vi "8HP_Channels.vi"(1 "Analysis Info cluster":T2[](array[typedef]) {"Sync Delay Time (s)" format="%.4f"; "Sd Error in Variance" format="%.2f"; "Skew_u" format="%.2f"; "% u'/U" format="%.2f"; "Sd Error in Mean" format="%.2f"; "Kurt_u" format="%.2f"; "u^4" format="%.2f"; "u^3" format="%.2f"; "U" format="%.2f"; "u^2" format="%.2f"}) -> (0 "8HP Info":T1(array[cluster]))   [LabVIEW 2018]
uses:
  Controls/Analysis_info_cluster.ctl
  Controls/Inst_type.ctl
  Controls/Instrument_Array.ctl
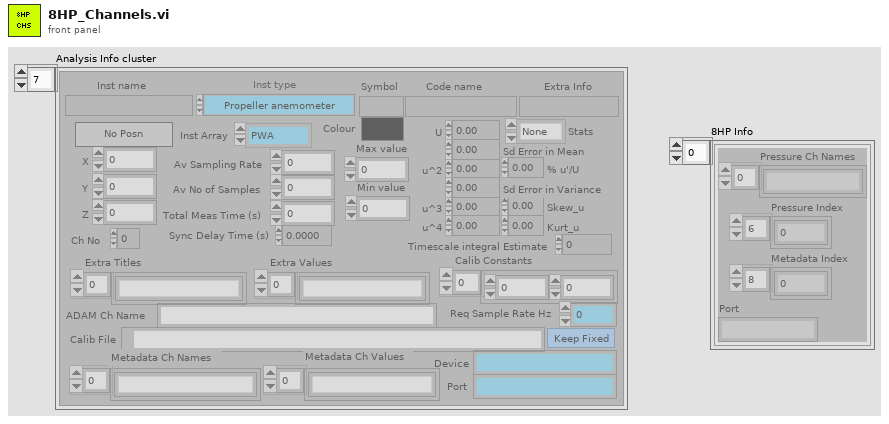
[diagram p1: front panel]
types:
  T1 = cluster{"Pressure Ch Names":string[], "Pressure Index":i32[], "Metadata Index":i32[], "Port":string}[]
  T2 = typedef "Analysis_info_cluster.ctl" = cluster{"Colour":u32, "Inst type":T3, "Inst name":string, "Symbol":string, "Code name":string, "Extra Info":string, "Inst Array":T4, "Extra Titles":string[], "Extra Values":string[], "U":dbl, "u^2":dbl, "u^3":dbl, "u^4":dbl, "Skew_u":dbl, "Kurt_u":dbl, "Sd Error in Mean":dbl, "% u'/U":dbl, "X":dbl, "Y":dbl, "Z":dbl, "Timescale integral Estimate":dbl, "Sd Error in Variance":dbl, "Calib File":path, "Calib Constants":dbl[], "Output Position":bool, "Stats":enum16{"None", "Basic", "Full"}, "Av Sampling Rate":dbl, "Av No of Samples":dbl, "Total Meas Time (s)":dbl, "ADAM Ch Name":string, "Max value":dbl, "Min value":dbl, "Req Sample Rate Hz":dbl, "Sync Delay Time (s)":dbl, "Ch No":i16, "Device":string, "Use Latest Calib":bool, "Port":string, "Metadata Ch Names":string[], "Metadata Ch Values":string[]}
  T3 = typedef "Inst_type.ctl" = enum16{"Propeller anemometer", "Raw voltage", "Pressure Transducer", "Pitot-static tube", "Preston tube", "Hot wire", "Cross wire 1", "Cross wire 2", "Generic Linear", "Generic Polynomial", "Generic BackPoly", "Fast FID", "Thermocouple", "Cold wire", "Pulsed Wire", "LDA Vel", "LDA Tran time", "LDA Arr time", "Microphone"}
  T4 = typedef "Instrument_Array.ctl" = enum16{"PWA", "LDA", "Analogue"}
  T5 = cluster{"Pressure Ch Names":string[], "Pressure Index":i32[], "Metadata Index":i32[], "Port":string}
  T6 = typedef "Device ID port info.ctl" = cluster{"Ch No":i16[], "Req Sampling Rate":dbl[], "Port":string, "Index":i32[]}
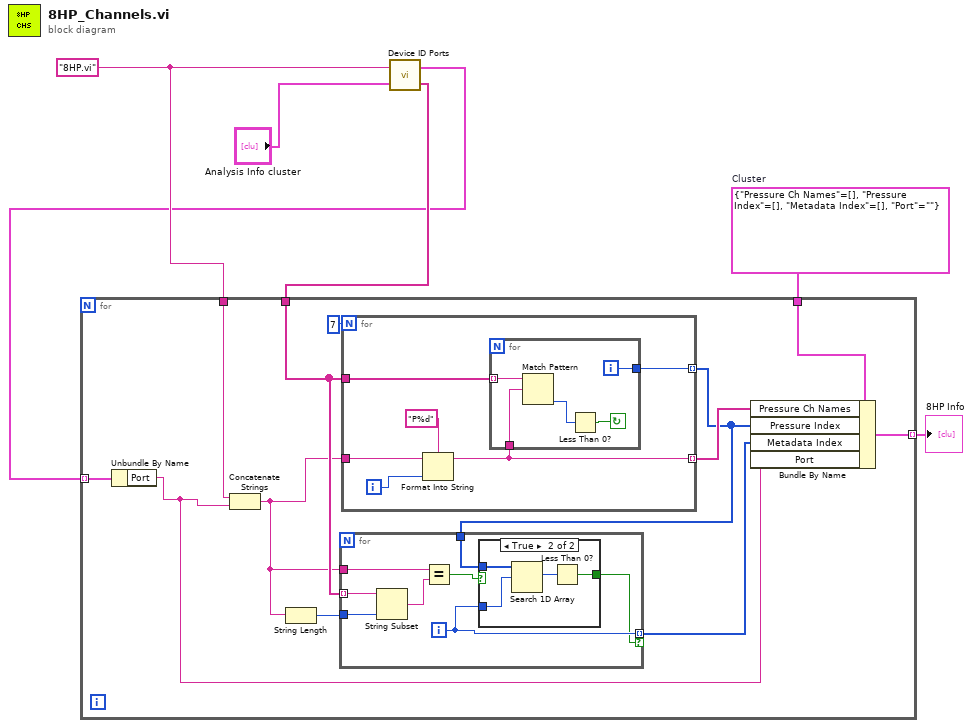
[diagram p0: block diagram]
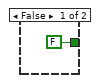
[diagram p2: hidden frame]
diagram:
  w3 = T5 {"Pressure Ch Names"=[], "Pressure Index"=[], "Metadata Index"=[], "Port"=""}  # Cluster
  w5 = "8HP.vi" ("Device ID")
  n1 = call "Device ID Ports.vi"("Analysis Info cluster"="Analysis Info cluster", "Device ID"=w5) -> ("Unique Channel Names"=w4:string[], "Device port info"=w1:T6[])
  n2 = for {
    tunnel: w5 -> [w18]
    tunnel: w4 -> [w13]
    tunnel: w3 -> [w16]
    tunnel: [w9] -> w2 mode=indexing
    tunnel: w1 -> [w8] mode=indexing
    n3 = Unbundle By Name(w8) -> ("Port"=w7:string)
    n4 = Concatenate Strings(w18, w7) -> (w12:string)
    n5 = String Length(string=w12) -> (length=w14:i32)
    n6 = for {
      N: 7 -> [_]
      tunnel: w13 -> [w35]
      tunnel: [w34] -> w11 mode=indexing
      tunnel: w12 -> [w33]
      tunnel: [w32] -> w15 mode=indexing
      i -> [w37]
      n7 = Format Into String(format string="P%d", initial string=w33, w37) -> (resulting string=w32:string)  [unwired: 1 in, 1 out]
      n8 = for {
        tunnel: w35 -> [w38] mode=indexing
        tunnel: w32 -> [w42]
        tunnel: [w39] -> w34
        i -> [w39]
        stop <- w41 continue-if-true
        n9 = Match Pattern(string=w38, regular expression=w42) -> (offset past match=w40:i32)  [unwired: 1 in, 3 out]
        n10 = Less Than 0?(x=w40) -> (x < 0?=w41:bool)
      }
    }
    n11 = for {
      tunnel: w14 -> [w26]
      tunnel: w13 -> [w25] mode=indexing
      tunnel: w12 -> [w23]
      tunnel: w11 -> [w21]
      tunnel: [w20] -> w10 mode=indexing if=w19
      i -> [w20]
      n12 = String Subset(string=w25, length (rest)=w26) -> (substring=w24:string)  [unwired: 1 in]
      n13 = Equal?(x=w23, y=w24) -> (x = y?=w22:bool)
      n14 = case shown="True" w22 {
        tunnel: w21 -> [_ w31]
        tunnel: w20 -> [_ w30]
        tunnel: [FALSE w28] -> w19
        frame False {
        }
        frame True {
          n15 = Search 1D Array(1D array=w31, element=w30) -> (index of element=w29:i32)  [unwired: 1 in]
          n16 = Less Than 0?(x=w29) -> (x < 0?=w28:bool)
        }
      }
    }
    n17 = Bundle By Name(cluster=w16, "Pressure Ch Names"=w15, "Pressure Index"=w11, "Metadata Index"=w10, "Port"=w7) -> (w9:T5)
  }
  "8HP Info" <- w2
